vi "Navigating Hierarchy Example with VI Scripting.vi"() -> ()   [LabVIEW 2026]
panel:
  out "error out":errorcluster
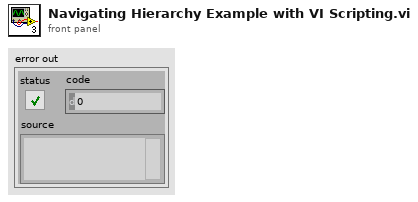
[diagram p1: front panel]
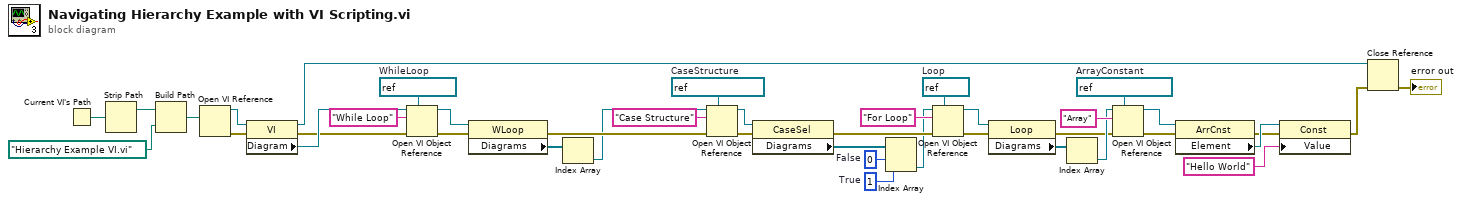
[diagram p0: block diagram]
diagram:
  w14 = refnum<vi> refnum  # ArrayConstant
  w18 = 1  # True
  w19 = 0  # False
  w22 = refnum<vi> refnum  # Loop
  w32 = refnum<vi> refnum  # CaseStructure
  w34 = refnum<vi> refnum  # WhileLoop
  n1 = Current VI's Path() -> (path=w4:path)
  n2 = Strip Path(path=w4) -> (stripped path=w3:path)  [unwired: 1 out]
  n3 = Build Path(base path=w3, name or relative path=path "Hierarchy Example VI.vi") -> (appended path=w1:path)
  n4 = Open VI Reference(vi path=w1) -> (vi reference=w41:refnum<vi>, error out=w40:errorcluster)  [unwired: 5 in]
  n5 = property class="VI"(reference=w41, error in=w40) -> (reference out=w36:refnum<vi>, error out=w38:errorcluster, "Diagram"=w39:refnum<vi>)
  n6 = Open VI Object Reference(7:w34, 8:w38, 10:"While Loop" ("name/order"), 11:w39) -> (0:w31:errorcluster, 3:w29:refnum<vi>)
  n7 = property class="WLoop"(reference=w29, error in=w31) -> (error out=w30:errorcluster, "Diagrams"=w28:refnum<vi>[])  [unwired: 1 out]
  n8 = Index Array(array=w28) -> (element=w27:refnum<vi>)  [unwired: 1 in]
  n9 = Open VI Object Reference(7:w32, 8:w30, 10:"Case Structure" ("name/order"), 11:w27) -> (0:w25:errorcluster, 3:w26:refnum<vi>)
  n10 = property class="CaseSel"(reference=w26, error in=w25) -> (error out=w21:errorcluster, "Diagrams"=w24:refnum<vi>[])  [unwired: 1 out]
  n11 = Index Array(array=w24, index #1=w19, index #2=w18) -> (element #2=w20:refnum<vi>)  [unwired: 1 out]
  n12 = Open VI Object Reference(7:w22, 8:w21, 10:"For Loop" ("name/order"), 11:w20) -> (0:w16:errorcluster, 3:w17:refnum<vi>)
  n13 = property class="Loop"(reference=w17, error in=w16) -> (error out=w11:errorcluster, "Diagrams"=w13:refnum<vi>[])  [unwired: 1 out]
  n14 = Index Array(array=w13) -> (element=w12:refnum<vi>)  [unwired: 1 in]
  n15 = Open VI Object Reference(7:w14, 8:w11, 10:"Array" ("name/order"), 11:w12) -> (0:w9:errorcluster, 3:w10:refnum<vi>)
  n16 = property class="ArrCnst"(reference=w10, error in=w9) -> (error out=w7:errorcluster, "Element"=w8:refnum<vi>)  [unwired: 1 out]
  n17 = property class="Const"(reference=w8, error in=w7, "Value"="Hello World") -> (error out=w6:errorcluster)  [unwired: 1 out]
  n18 = Close Reference(reference=w36, error in (no error)=w6) -> (error out=→"error out":errorcluster)
